vi "Decompile.vi"() -> ()   [LabVIEW 2011]
panel:
  out "lo(x)":u8
  out "hi(x) 3":u8
  out "hi(x) 2":u16
  in  "Array in":u8[](array[numeric])=[65, 32, 43, 48, 48, 48, 48, 46, 48, 32, 48, 48, 48, 48, 46, 48, 32, 13, 0, 65, 32, 43, 48, 48, 48, 48, 46, 48, 32, 48, 48, 48, 48, 46, 48, 32, 13, 0, 0, 0, 0, 0, 0, 0, 0, 0, 0, 0, 0, 0, 0, 0, 0, 0, 0, 0, 0, 0, 0, 0]
  out "Numeric":u64
  out "Array out":u32[](array[numeric])
  out "hi(x)":u32
  out "Array":u32[][](array[numeric])
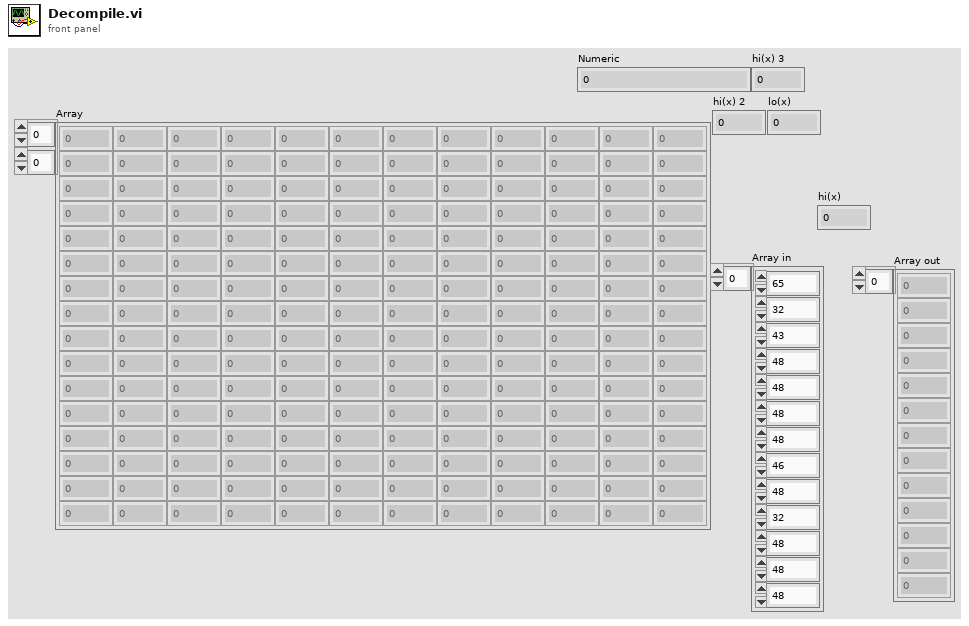
[diagram p1: front panel]
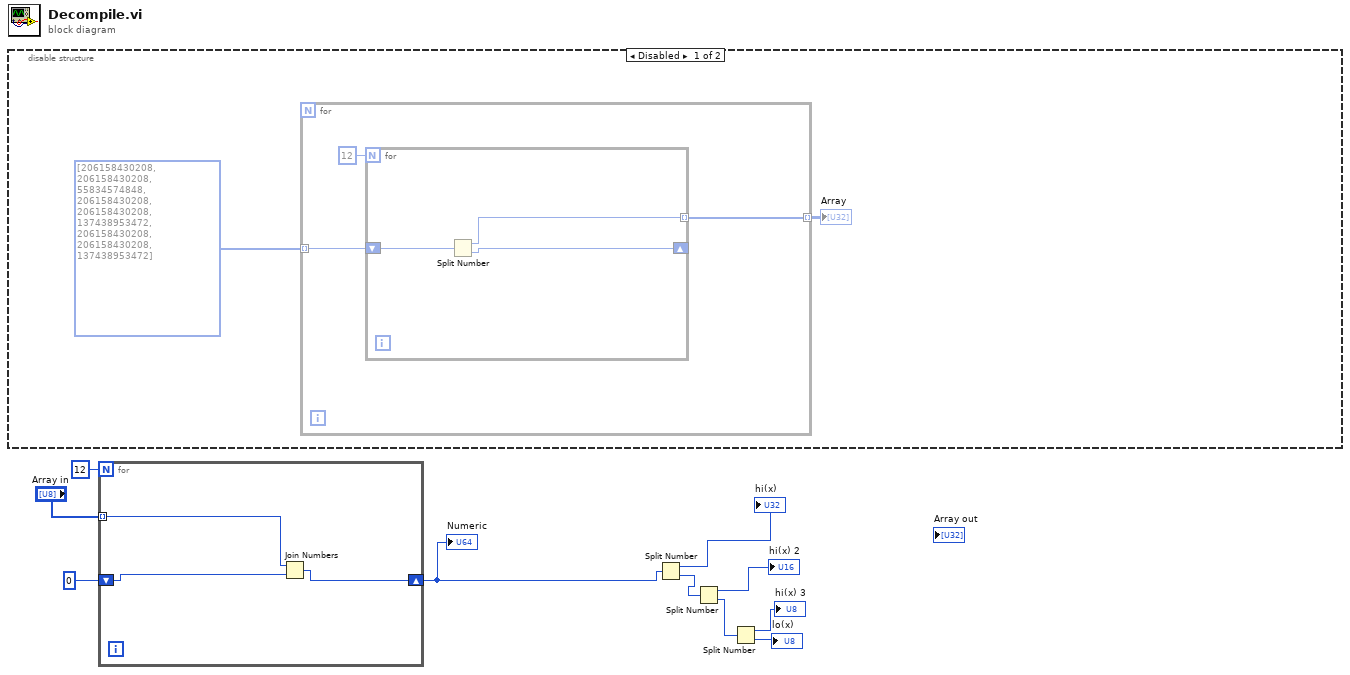
[diagram p0: block diagram]
diagram:
  n1 = disable-structure shown="Disabled" {
    frame Disabled {
      n2 = for {
        tunnel: u64[] [206158430208, 206158430208, 55834574848, 206158430208, 206158430208, 137438953472, 206158430208, 206158430208, 137438953472] ("MFC PV1") -> [w15] mode=indexing
        tunnel: [w13] -> w11 mode=indexing
        n3 = for {
          N: 12 -> [_]
          shift-right: [w17] -> _
          shift-left: w15 -> [w18]
          tunnel: [w16] -> w13 mode=indexing
          n4 = Split Number(x=w18) -> (hi(x)=w16:u32, lo(x)=w17:u32)
        }
      }
      "Array" <- w11
    }
    frame Enabled {
    }
  }
  n5 = for {
    N: 12 -> [_]
    shift-right: [w20] -> w6
    shift-left: 0 -> [w21]
    tunnel: "Array in" -> [w19] mode=indexing
    n6 = Join Numbers(hi=w19, lo=w21) -> ((hi.lo)=w20:u64)
  }
  "Numeric" <- w6
  n7 = Split Number(x=w6) -> (hi(x)=→"hi(x)":u32, lo(x)=w5:u32)
  n8 = Split Number(x=w5) -> (hi(x)=→"hi(x) 2":u16, lo(x)=w3:u16)
  n9 = Split Number(x=w3) -> (hi(x)=→"hi(x) 3":u8, lo(x)=→"lo(x)":u8)
